vi "Exercises AM Modulation.vi"(8 "基带幅度":dbl(slide) scale=0.0..200.0 scale format="%#_6p", 9 "基带频率":dbl(slide) scale=0.0..2000.0 scale format="%#_6p", 10 "载波幅度":dbl(slide) scale=0.0..1000.0 scale format="%#_6p", 11 "载波频率":dbl(slide) scale=0.0..20000.0 scale format="%#_6p") -> (2 "AM 调制信号 (时域)":waveform(dbl)(graph), 3 "载波信号":waveform(dbl)(graph))   [LabVIEW 2015]
uses:
  <vilib>/measure/NI_MABase.lvlib
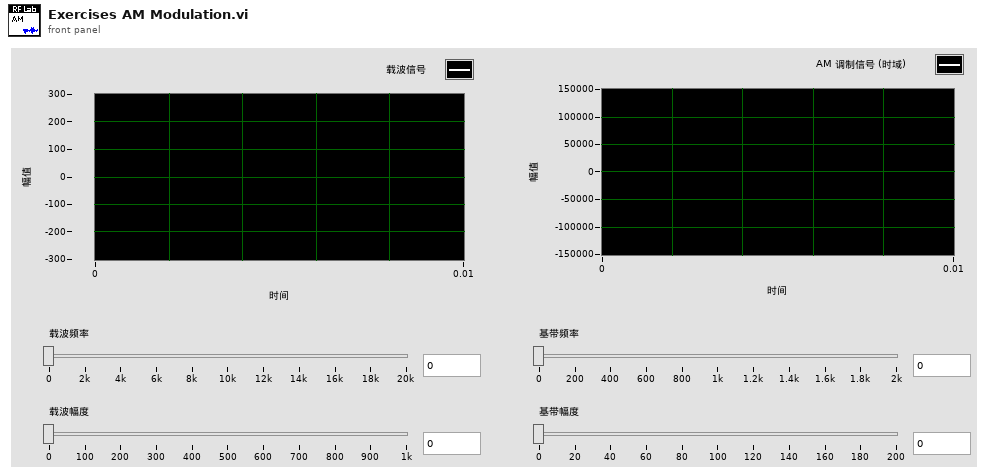
[diagram p1: front panel]
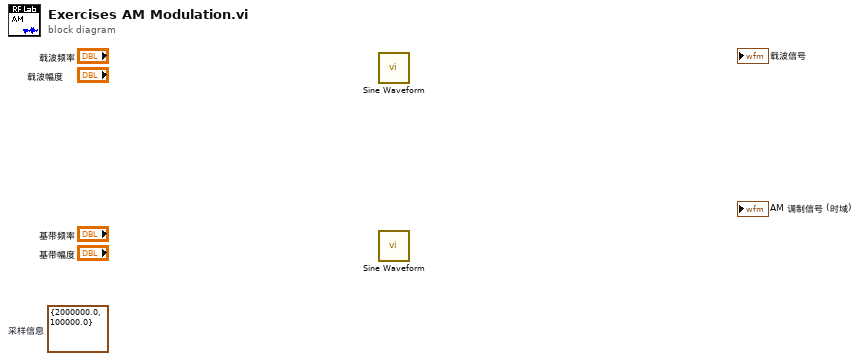
[diagram p0: block diagram]
diagram:
  (unwired) cluster{"Fs":dbl, "#s":dbl} {"Fs"=2000000.0, "#s"=100000.0}  # 采样信息
  n1 = call <vilib>:"Sine Waveform.vi"() -> ()  [unwired: 10 in, 2 out]
  n2 = call <vilib>:"Sine Waveform.vi"() -> ()  [unwired: 10 in, 2 out]
